vi "BRig_RT__Case_Exp__State_Reward.vi"(0 "input_dataCurrent":u16[](array[numeric]), 1 "input_state":T1, 9 "input_dataExp":u16[](array[numeric])) -> (3 "output_state":T1, 4 "output_dataCurrent":u16[](array[numeric]), 10 "output__L":bool, 15 "output__R":bool)   [LabVIEW 2014]
uses:
  myRIO_BRig_RT__Case_Exp_stateList.ctl
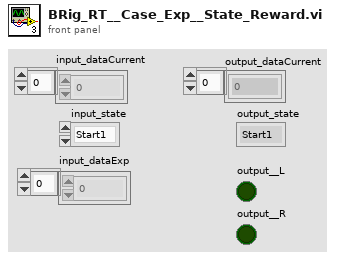
[diagram p1: front panel]
types:
  T1 = typedef "myRIO_BRig_RT__Case_Exp_stateList.ctl" = enum16{"Start1", "Start2", "Start3", "saveSettings1", "saveSettings2", "saveSettings3", "saveSettings4", "saveSettings_LC_ENL_l1", "saveSettings_LC_ENL_l2", "saveSettings_LC_Cue_l1", "saveSettings_LC_Cue_l2", "saveSettings6_LC_l1_Other", "SaveSettings6_LC_l2_Other", "setSettings_Audio", "setSettings_Laser", "initBlock_pre", "initBlock", "initBlock2", "initBlock_post", "initTrial_pre", "initTrial", "initTrial2", "initTrial3", "initTrial4", "initTrial_LC_ENL1", "initTrial_LC_Cue1", "initTrial_LC_Cue1_2", "initTrial_LC_Sel", "initTrial_post", "ENL1_pre", "ENL1", "ENL1_post", "ENL1Penalty_pre", "ENL1Penalty", "ENL2_pre", "ENL2", "ENL2Penalty_pre", "ENL2Penalty", "Cue1_pre", "Cue1", "Cue1_post", "Cue1Penalty_pre", "Cue1Penalty", "Cue2_pre", "Cue2", "Cue2Penalty_pre", "Cue2Penalty", "Selection_pre", "Selection", "Select_post", "SelectReward_pre", "SelectReward", "SelectRewardPost_pre", "SelectRewardPost", "SelectWrong_pre", "SelectWrong", "SelectWrong_post", "SelectTimeout_pre", "SelectTimeout", "SelectTimeout_post", "endTrial_pre", "endTrial1", "endTrial2", "endTrial3", "endTrial_post", "endBlock_pre", "endBlock", "endBlock_post", "endExp", "commConnect", "commUpload_pre", "commUpload_dataBlock", "commUpload_dataCurrent", "commUpload_dataExp", "commUpload_dataLC", "commUpload_dataTrial", "commUpload_post", "saveData_pre", "saveData_dataBlock", "saveData_dataCurrent", "saveData_dataExp", "saveData_dataLC", "saveData_dataTrial", "saveData_post", "empty_endBlock1", "empty_endBlock2", "empty_endTrial1", "empty_endTrial2", "empty_endTrial3", "empty_endTrial4", "empty_endTrial5", "dummyState", "dummyState_endBlock", "FreeReward_pre", "FreeReward", "FreeRewardPost_pre", "FreeRewardPost"}
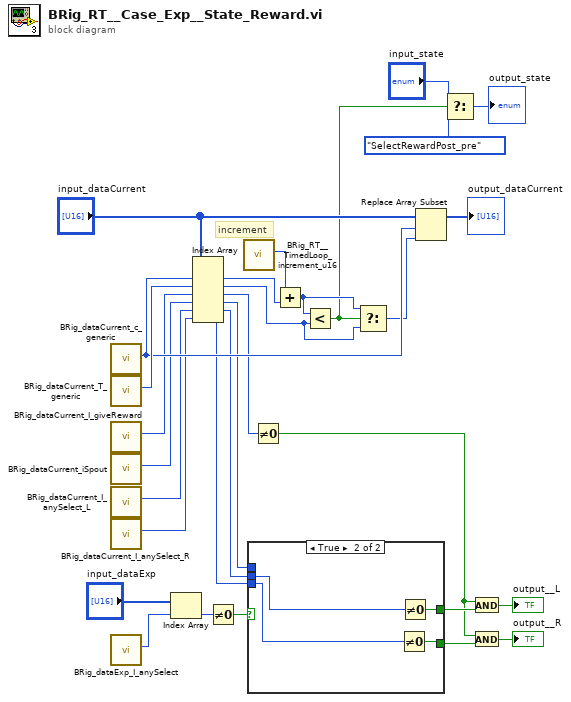
[diagram p0: block diagram]
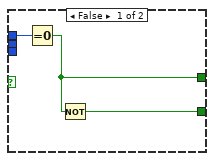
[diagram p2: hidden frame]
diagram:
  # "increment"
  n1 = call "BRig_dataCurrent_c_generic.vi"() -> ("output_count_generic"=w26:i32)  [unwired: 11 in]
  n2 = call "BRig_dataCurrent_T_generic.vi"() -> ("output_T_generic"=w28:i32)  [unwired: 11 in]
  n3 = call "BRig_dataCurrent_I_giveReward.vi"() -> ("output_I_giveReward"=w17:i32)  [unwired: 11 in]
  n4 = call "BRig_dataCurrent_iSpout.vi"() -> ("output_iSpout"=w7:i32)  [unwired: 11 in]
  n5 = call "BRig_dataCurrent_I_anySelect_L.vi"() -> ("output_IanySelect_L"=w3:i32)  [unwired: 11 in]
  n6 = call "BRig_dataCurrent_I_anySelect_R.vi"() -> ("output_IanySelect_R"=w2:i32)  [unwired: 11 in]
  n7 = call "BRig_dataExp_I_anySelect.vi"() -> ("output_I_anySelect"=w13:i32)  [unwired: 11 in]
  n8 = Index Array(array="input_dataExp", index=w13) -> (element=w12:u16)
  n9 = Index Array(array="input_dataCurrent", index #1=w26, index #2=w28, index #3=w17, index #4=w7, index #5=w3, index #6=w2) -> (element #1=w27:u16, element #2=w25:u16, element #3=w8:u16, element #4=w6:u16, element #5=w5:u16, element #6=w1:u16)
  n10 = Not Equal To 0?(x=w12) -> (x != 0?=w11:bool)
  n11 = call "BRig_RT__TimedLoop_increment_u16.vi"() -> ("output_increment__u16"=w23:u16)  [unwired: 11 in]
  n12 = case shown="True" w11 {
    tunnel: [w31 w37] -> w10
    tunnel: [w33 w36] -> w9
    tunnel: w6 -> [w32 _]
    tunnel: w5 -> [_ w35]
    tunnel: w1 -> [_ w34]
    frame False {
      n13 = Equal To 0?(x=w32) -> (x = 0?=w31:bool)
      n14 = Not(x=w31) -> (.not. x?=w33:bool)
    }
    frame True {
      n15 = Not Equal To 0?(x=w34) -> (x != 0?=w36:bool)
      n16 = Not Equal To 0?(x=w35) -> (x != 0?=w37:bool)
    }
  }
  n17 = Not Equal To 0?(x=w8) -> (x != 0?=w4:bool)
  n18 = Add(x=w23, y=w27) -> (x+y=w22:u16)
  n19 = Less?(x=w22, y=w25) -> (x < y?=w18:bool)
  n20 = Select(t=w22, s=w18, f=w25) -> (s? t:f=w24:u16)
  n21 = Replace Array Subset(array="input_dataCurrent", new element=w24, index=w26) -> (→"output_dataCurrent":u16[])
  n22 = Select(t="input_state", s=w18, f=myRIO_BRig_RT__Case_Exp_stateList."SelectRewardPost_pre" ("Enum")) -> (s? t:f=→"output_state":T1)
  n23 = And(x=w4, y=w10) -> (x .and. y?=→"output__L":bool)
  n24 = And(x=w4, y=w9) -> (x .and. y?=→"output__R":bool)
